vi "Test Assert Valid Refnum.vi"(8 "error in (no error)":errorcluster) -> (0 "error out":errorcluster)   [LabVIEW 2013]
uses:
  classes/Assert/Assert.lvclass
  classes/Test/Test.lvclass
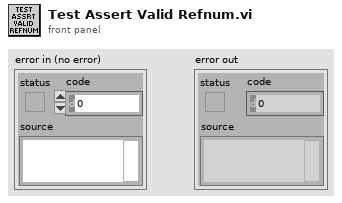
[diagram p1: front panel]
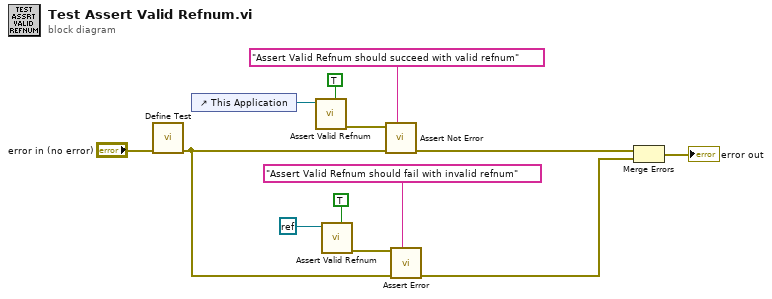
[diagram p0: block diagram]
diagram:
  n1 = call "Define Test.vi"("error in (no error)"="error in (no error)") -> ("error out"=w3:errorcluster)  [unwired: 9 in, 1 out]
  n2 = control-ref of="This Application"() -> (w2:refnum<vi>)
  n3 = call "Assert Valid Refnum.vi"("Assert Only? (F)"=TRUE, "Refnum"=w2) -> ("error out"=w13:errorcluster)  [unwired: 8 in, 1 out]
  n4 = call "Assert Valid Refnum.vi"("Assert Only? (F)"=TRUE, "Refnum"=refnum<k0> refnum) -> ("error out"=w11:errorcluster)  [unwired: 8 in, 1 out]
  n5 = call "Assert Not Error.vi"("Label"="Assert Valid Refnum should succeed with valid refnum", "error in (no error)"=w3, "Not Error?"=w13) -> ("error out"=w5:errorcluster)  [unwired: 7 in, 1 out]
  n6 = call "Assert Error.vi"("Label"="Assert Valid Refnum should fail with invalid refnum", "error in (no error)"=w3, "Error?"=w11) -> ("error out"=w6:errorcluster)  [unwired: 7 in, 1 out]
  n7 = Merge Errors(w5, w6) -> (→"error out":errorcluster)
